vi "ClsGetLastSampleSingleChannelDevice.vi"(8 "error in (no error)":errorcluster, 11 "Connection In":u32) -> (0 "error out":errorcluster, 2 "Data":dbl[](array[numeric]), 3 "Connection Out":u32, 5 "Have data?":bool)   [LabVIEW 2010]
doc: "Get Last Sample:\n\nThis function is especially targeted for single channel devices. This function is used to get the last/newest valid sample from device(which may be duplicated for several consecutive calls if no newer sample is available). By calling this function, client will also jump to the last valid position in the data buffer used to temporarily store the data from device. Note that this function is none-block which means it will return immediately no matter if there is any data available.\n\nConnection In[Input]: the connection handle which is initially created by Open Connection subVI.\n\nHave data?[Output]: since this subVI is none-block which will return immediately with an empty data array if there is no data available, this boolean output is used for indicating whether there is any data in the output at all.\n\nData[Output]: The one dimensional array for data. Note that you can use Get Signal IDs subVI to see the ordering of signal IDs correspondent to this data array. If there is no data, an empty array will be returned.\n\nConnection Out[Output]: the connection handle output which could be used for next subVI refering to the same connection."
uses:
  dependent dlls/CHRocodileDLL.dll
panel:
  out "_pnNumberOfSignals":i32
  out "return type":i32
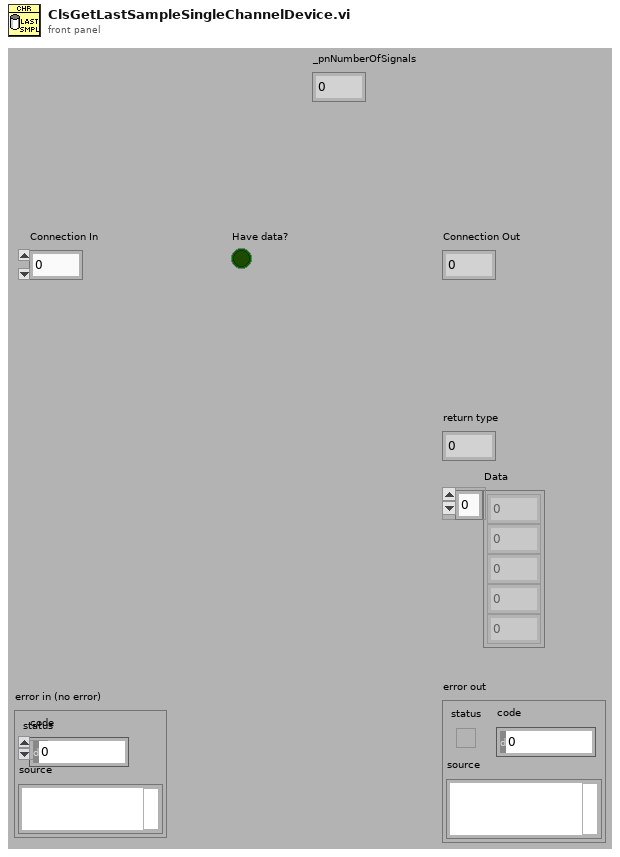
[diagram p1: front panel]
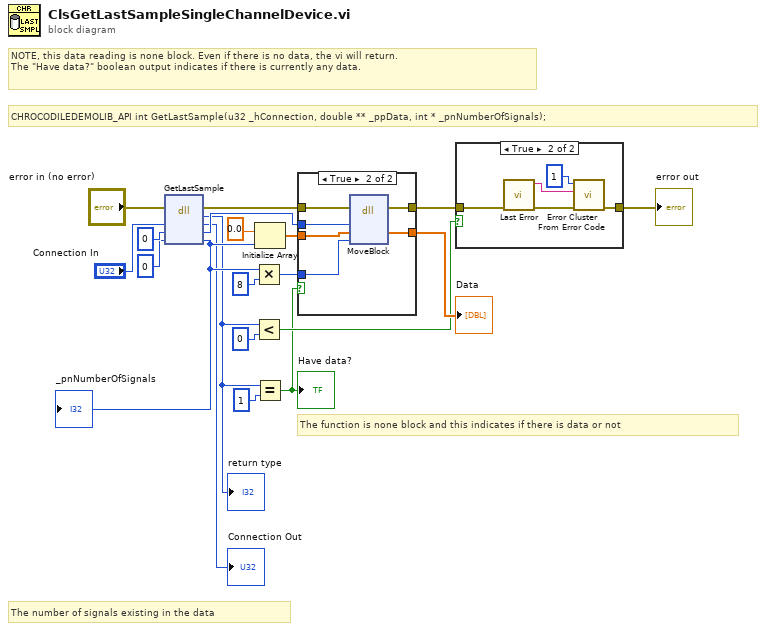
[diagram p0: block diagram]
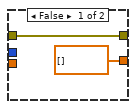
[diagram p2: hidden frame]
diagram:
  # "The function is none block and this indicates if there is data or not"
  # "The number of signals existing in the data"
  # "NOTE, this data reading is none block. Even if there is no data, the vi will return.\nThe \"Have data?\" boolean output indicates if there is currently any data."
  # "CHROCODILEDEMOLIB_API int GetLastSample(u32 _hConnection, double ** _ppData, int * _pnNumberOfSignals);"
  n1 = dll-call lib="C:/Users/y.ji/Desktop/CHRocodile VIs 1.0/dependent dlls/CHRocodileDLL.dll" fn="GetLastSample"(error in="error in (no error)", "_hConnection"="Connection In", "_ppData"=i64 0, "_pnNumberOfSignals"=i64 0) -> (error out=w11:errorcluster, "return type"=w5:i32, "_hConnection"=→"Connection Out":u32, "_ppData"=w19:i64, "_pnNumberOfSignals"=w15:i32)  [unwired: 2 in, 1 out]
  "return type" <- w5
  "_pnNumberOfSignals" <- w15
  n2 = Multiply(x=w15, y=8) -> (x*y=w17:i32)
  n3 = Less?(x=w5, y=0) -> (x < y?=w7:bool)
  n4 = Initialize Array(0.0, w15) -> (w14:dbl[])
  n5 = Equal?(x=w5, y=1) -> (x = y?=w1:bool)
  "Have data?" <- w1
  n6 = case shown="True" w1 {
    tunnel: w19 -> [_ w28]
    tunnel: w17 -> [_ w27]
    tunnel: w14 -> [_ w26]
    tunnel: [dbl[] [] ("Destination") w25] -> w13
    tunnel: w11 -> [w21 w24]
    tunnel: [w21 w23] -> w6
    frame False {
    }
    frame True {
      n7 = dll-call lib="LabVIEW" fn="MoveBlock"(error in=w24, "Address(pointer)"=w28, "Destination"=w26, "Size"=w27) -> (error out=w23:errorcluster, "Destination"=w25:dbl[])  [unwired: 5 in, 1 out]
    }
  }
  "Data" <- w13
  n8 = case shown="True" w7 {
    tunnel: [w29 w33] -> w9
    tunnel: w6 -> [w29 w30]
    frame False {
    }
    frame True {
      n9 = call "Last Error.vi"("error in (no error)"=w30) -> ("error out"=w31:errorcluster, "Error Message"=w32:string)  [unwired: 9 in]
      n10 = call <vilib>:"Error Cluster From Error Code.vi"("error in (no error)"=w31, "error message (\"\")"=w32, "error code (0)"=1) -> ("error out"=w33:errorcluster)  [unwired: 6 in]
    }
  }
  "error out" <- w9
